vi "Define Name.vi"(8 "error in":errorcluster, 11 "module in":refnum<class "Module.lvclass">) -> (0 "error out":errorcluster, 3 "module out":refnum<class "Module.lvclass">)   [LabVIEW 2020, in "Scan Engine Scripting.lvlib" / "Module.lvclass"]
uses:
  Module.lvclass
  <vilib>/regexp/Match Regular Expression.xnode
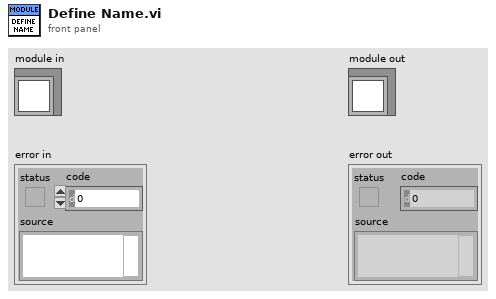
[diagram p1: front panel]
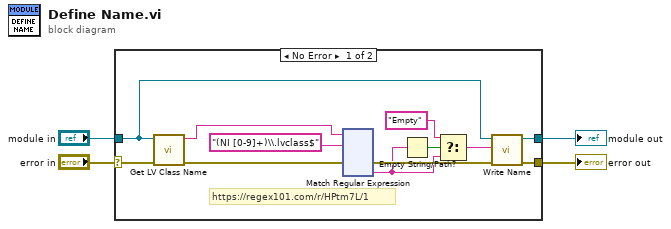
[diagram p0: block diagram]
diagram:
  n1 = case shown="No Error" "error in" {
    selector: "error in" -> [w16 w134]
    tunnel: [w9 w134] -> w3
    tunnel: [w11 w133] -> w1
    tunnel: "module in" -> [w12 w133]
    frame No Error {
      # "https://regex101.com/r/HPtm7L/1"
      n2 = call <vilib>:"Get LV Class Name.vi"("error in (no error)"=w16, "object"=w12) -> ("error out"=w13:errorcluster, "class name"=w14:string)  [unwired: 8 in]
      n3 = xnode "Match Regular Expression"("input string"=w14, "regular expression"="(NI [0-9]+)\\.lvclass$", "error in"=w13) -> ("error out"=w10:errorcluster, "submatch 1"=w5:string)  [unwired: 3 in, 4 out]
      n4 = Empty String/Path?(string/path=w5) -> (empty?=w8:bool)
      n5 = Select(t="Empty", s=w8, f=w5) -> (s? t:f=w6:string)
      n6 = call-dynamic "Write Name.vi"("error in"=w10, "name"=w6, "module in"=w12) -> ("error out"=w9:errorcluster, "module out"=w11:refnum<class "Module.lvclass">)  [unwired: 7 in]
    }
    frame Error {
    }
  }
  "error out" <- w3
  "module out" <- w1
